vi "Format Dictionary.vi"(7 "error in (no error)":errorcluster, 9 "Measurement Parameters In":refnum<class "String Database.lvclass">, 10 "QPA TCF Parser in":refnum<class "QPA TCF Parser.lvclass">) -> (0 "error out":errorcluster, 2 "String Database out":refnum<class "String Database.lvclass">)   [LabVIEW 2016, in "QPA TCF Parser.lvlib" / "QPA TCF Parser.lvclass"]
uses:
  QPA TCF Parser.lvclass
  Plugins/String Database.lvlibp/String Database.lvclass
panel:
  out "QPA TCF Parser out":refnum<class "QPA TCF Parser.lvclass">
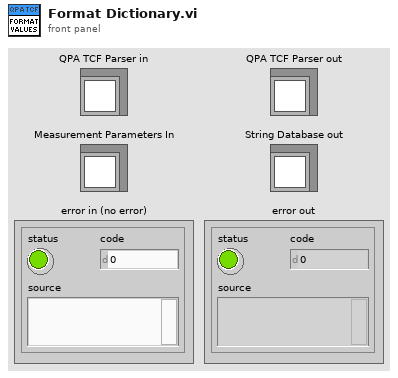
[diagram p1: front panel]
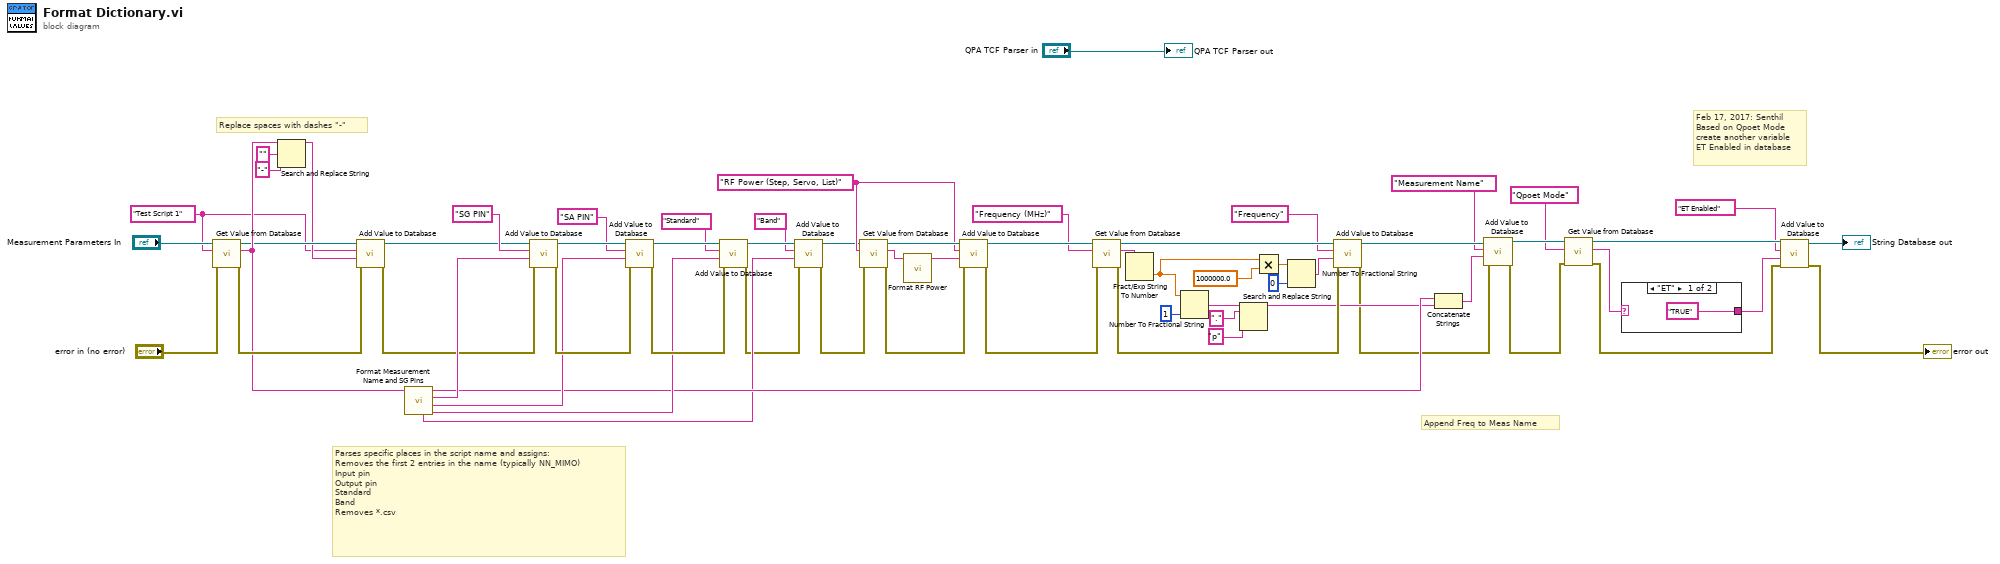
[diagram p0: block diagram]
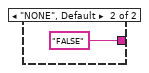
[diagram p2: hidden frame]
diagram:
  w58 = "RF Power (Step, Servo, List)" ("Entry Name")
  w30 = "Test Script 1" ("Entry Name")
  # "Feb 17, 2017: Senthil\nBased on Qpoet Mode \ncreate another variable\nET Enabled in database"
  # "Parses specific places in the script name and assigns:\nRemoves the first 2 entries in the name (typically NN_MIMO)\nInput pin\nOutput pin\nStandard\nBand\nRemoves *.csv"
  # "Append Freq to Meas Name"
  # "Replace spaces with dashes \"-\""
  n1 = call "Get Value from Database.vi"("error in (no error)"="error in (no error)", "Entry Name"=w30, "Message in"="Measurement Parameters In") -> ("error out"=w56:errorcluster, "Entry Value"=w37:string, "Message out"=w33:refnum<class "String Database.lvclass">)  [unwired: 5 in, 1 out]
  n2 = Search and Replace String(input string=w37, search string="-", replace string="" ("replace string (\"\")")) -> (result string=w31:string)  [unwired: 5 in, 3 out]
  n3 = call "Add Value to Database.vi"("error in (no error)"=w56, "Entry Value"=w31, "Entry Name"=w30, "Dictionary In"=w33) -> ("error out"=w34:errorcluster, "Dictionary Out"=w32:refnum<class "String Database.lvclass">)  [unwired: 5 in, 1 out]
  n4 = call "Format Measurement Name and SG Pins.vi"("Test Script In"=w37) -> ("Standard"=w45:string, "SA Pin"=w50:string, "SG Pin"=w52:string, "Measurement Name Out"=w26:string, "Band"=w14:string)  [unwired: 6 in]
  n5 = call "Add Value to Database.vi"("error in (no error)"=w34, "Entry Value"=w52, "Entry Name"="SG PIN", "Dictionary In"=w32) -> ("error out"=w55:errorcluster, "Dictionary Out"=w53:refnum<class "String Database.lvclass">)  [unwired: 5 in, 1 out]
  n6 = call "Add Value to Database.vi"("error in (no error)"=w55, "Entry Value"=w50, "Entry Name"="SA PIN", "Dictionary In"=w53) -> ("error out"=w54:errorcluster, "Dictionary Out"=w47:refnum<class "String Database.lvclass">)  [unwired: 5 in, 1 out]
  n7 = call "Add Value to Database.vi"("error in (no error)"=w54, "Entry Value"=w45, "Entry Name"="Standard", "Dictionary In"=w47) -> ("error out"=w13:errorcluster, "Dictionary Out"=w17:refnum<class "String Database.lvclass">)  [unwired: 5 in, 1 out]
  n8 = call "Add Value to Database.vi"("error in (no error)"=w13, "Entry Value"=w14, "Entry Name"="Band", "Dictionary In"=w17) -> ("error out"=w12:errorcluster, "Dictionary Out"=w16:refnum<class "String Database.lvclass">)  [unwired: 5 in, 1 out]
  n9 = call "Get Value from Database.vi"("error in (no error)"=w12, "Entry Name"=w58, "Message in"=w16) -> ("error out"=w62:errorcluster, "Entry Value"=w61:string, "Message out"=w60:refnum<class "String Database.lvclass">)  [unwired: 5 in, 1 out]
  n10 = call "Format RF Power.vi"("RF Power In"=w61) -> ("Formatted RF Power"=w57:string)  [unwired: 10 in]
  n11 = call "Add Value to Database.vi"("error in (no error)"=w62, "Entry Value"=w57, "Entry Name"=w58, "Dictionary In"=w60) -> ("error out"=w48:errorcluster, "Dictionary Out"=w59:refnum<class "String Database.lvclass">)  [unwired: 5 in, 1 out]
  n12 = call "Get Value from Database.vi"("error in (no error)"=w48, "Entry Name"="Frequency (MHz)", "Message in"=w59) -> ("error out"=w44:errorcluster, "Entry Value"=w21:string, "Message out"=w40:refnum<class "String Database.lvclass">)  [unwired: 5 in, 1 out]
  n13 = Fract/Exp String To Number(string=w21) -> (number=w19:dbl)  [unwired: 3 in, 1 out]
  n14 = Number To Fractional String(number=w19, precision (6)=i16 1) -> (F-format string=w18:string)  [unwired: 2 in]
  n15 = Search and Replace String(input string=w18, search string=".", replace string="p" ("replace string (\"\")")) -> (result string=w25:string)  [unwired: 5 in, 3 out]
  n16 = Multiply(x=w19, y=1000000.0) -> (x*y=w41:dbl)
  n17 = Number To Fractional String(number=w41, precision (6)=i16 0) -> (F-format string=w39:string)  [unwired: 2 in]
  n18 = call "Add Value to Database.vi"("error in (no error)"=w44, "Entry Value"=w39, "Entry Name"="Frequency", "Dictionary In"=w40) -> ("error out"=w24:errorcluster, "Dictionary Out"=w23:refnum<class "String Database.lvclass">)  [unwired: 5 in, 1 out]
  n19 = Concatenate Strings(w26, w25) -> (w27:string)
  n20 = call "Add Value to Database.vi"("error in (no error)"=w24, "Entry Value"=w27, "Entry Name"="Measurement Name", "Dictionary In"=w23) -> ("error out"=w9:errorcluster, "Dictionary Out"=w10:refnum<class "String Database.lvclass">)  [unwired: 5 in, 1 out]
  n21 = call "Get Value from Database.vi"("error in (no error)"=w9, "Entry Name"="Qpoet Mode", "Message in"=w10) -> ("error out"=w3:errorcluster, "Entry Value"=w8:string, "Message out"=w6:refnum<class "String Database.lvclass">)  [unwired: 5 in, 1 out]
  n22 = case shown="\"ET\"" w8 {
    tunnel: ["TRUE" ("x") "FALSE" ("x")] -> w1
    frame "ET" {
    }
    frame "NONE", Default {
    }
  }
  n23 = call "Add Value to Database.vi"("error in (no error)"=w3, "Entry Value"=w1, "Entry Name"="ET Enabled", "Dictionary In"=w6) -> ("error out"=→"error out":errorcluster, "Dictionary Out"=→"String Database out":refnum<class "String Database.lvclass">)  [unwired: 5 in, 1 out]
  "QPA TCF Parser out" <- "QPA TCF Parser in"
